vi "toggle2.vi"() -> ()   [LabVIEW 2013]
panel:
  out "toggle on/off":bool
  in  "toggle on/off internal":bool
  in  "last switch":bool
  in  "current switch":bool
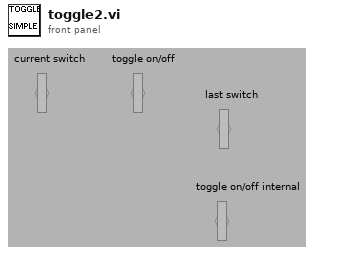
[diagram p1: front panel]
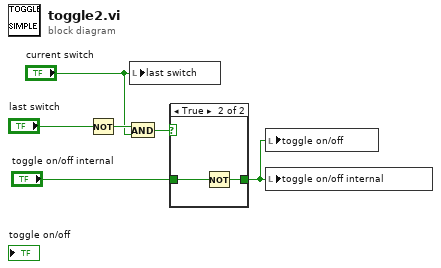
[diagram p0: block diagram]
diagram:
  n1 = Not(x="last switch") -> (.not. x?=w5:bool)
  n2 = And(x=w5, y="current switch") -> (x .and. y?=w4:bool)
  n3 = local write "last switch"("current switch") -> ()
  n4 = case shown="True" w4 {
    tunnel: "toggle on/off internal" -> [w7 w9]
    tunnel: [w7 w8] -> w2
    frame False {
    }
    frame True {
      n5 = Not(x=w9) -> (.not. x?=w8:bool)
    }
  }
  n6 = local write "toggle on/off"(w2) -> ()
  n7 = local write "toggle on/off internal"(w2) -> ()
